vi "Read.vi"(8 "error in (no error)":errorcluster, 11 "VeriStand DSF in":refnum<class "VeriStand Data Sharing Framework.lvclass">=refnum) -> (0 "error out":errorcluster, 3 "VeriStand DSF out":refnum<class "VeriStand Data Sharing Framework.lvclass">)   [LabVIEW 2017, in "Data Sharing Framework Engine.lvlib" / "VeriStand Data Sharing Framework.lvclass"]
uses:
  VeriStand Data Sharing Framework.lvclass
  DSF Core.lvlibp/Engine/Classes/Framework/Framework.lvclass
  C:/Git/DSF/VeriStand Data Sharing Custom Device/Data Sharing Custom Device/Source/Engine/DSF Core.lvlibp/Engine/Classes/Framework/Framework.lvclass
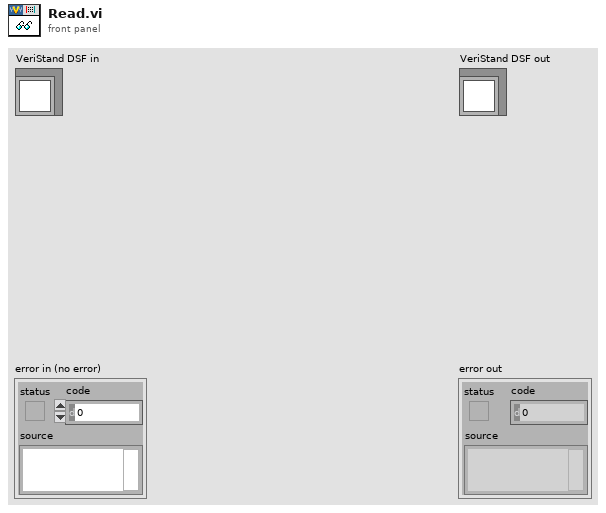
[diagram p1: front panel]
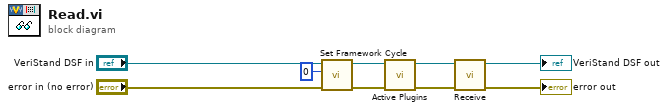
[diagram p0: block diagram]
diagram:
  n1 = call "Set Framework Cycle.vi"("error in (no error)"="error in (no error)", "iteration"=u64 0, "Framework in"="VeriStand DSF in") -> ("error out"=w6:errorcluster, "Framework out"=w7:refnum<class "VeriStand Data Sharing Framework.lvclass">)  [unwired: 7 in]
  n2 = call "Active Plugins.vi"("error in (no error)"=w6, "Framework in"=w7) -> ("error out"=w4:errorcluster, "Framework out"=w5:refnum<class "VeriStand Data Sharing Framework.lvclass">)  [unwired: 8 in]
  n3 = call "Receive.vi"("error in (no error)"=w4, "Framework in"=w5) -> ("error out"=→"error out":errorcluster, "Framework out"=→"VeriStand DSF out":refnum<class "VeriStand Data Sharing Framework.lvclass">)  [unwired: 8 in]
